vi "getChannelNumber.vi"(8 "error in (no error)":errorcluster, 11 "SoundAO in":refnum<class "SoundAO.lvclass">) -> (0 "error out":errorcluster, 2 "numberOfChannels":i32, 3 "SoundAO out":refnum<class "SoundAO.lvclass">)   [LabVIEW 2009, in "Hardware.lvlib" / "Channels.lvlib" / "SoundAO.lvclass"]
uses:
  SoundAO.lvclass
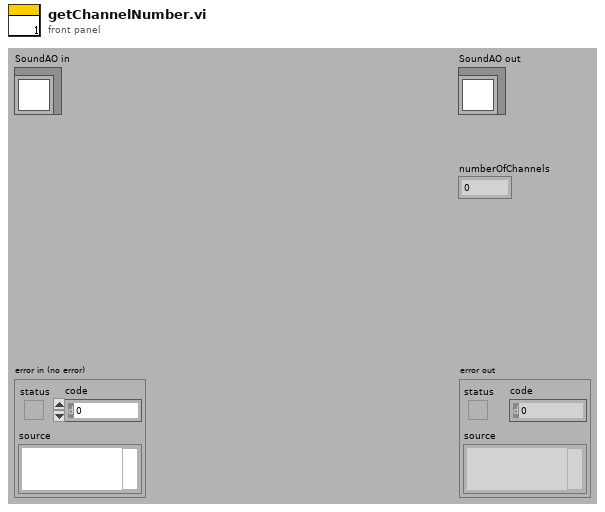
[diagram p1: front panel]
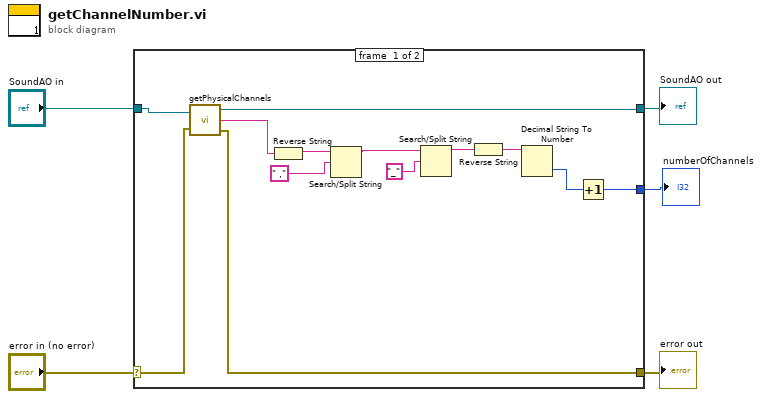
[diagram p0: block diagram]
diagram:
  n1 = case shown="No Error" "error in (no error)" {
    selector: "error in (no error)" -> [w17 w20]
    tunnel: [w15 w20] -> w4
    tunnel: [w16 w19] -> w2
    tunnel: "SoundAO in" -> [w18 w19]
    tunnel: [w6 _] -> w1
    frame #0 {
      n2 = call-dynamic "getPhysicalChannels.vi"("AnalogOutput.lvclass in"=w18, "error in (no error)"=w17) -> ("AnalogOutput.lvclass out"=w16:refnum<class "SoundAO.lvclass">, "Physical Channels"=w14:string, "error out"=w15:errorcluster)
      n3 = Reverse String(1:w14) -> (0:w13:string)
      n4 = Search/Split String(string=w13, search string/char (-)=" ,") -> (substring before match=w10:string)  [unwired: 1 in, 2 out]
      n5 = Search/Split String(string=w10, search string/char (-)="_") -> (substring before match=w7:string)  [unwired: 1 in, 2 out]
      n6 = Reverse String(1:w7) -> (0:w8:string)
      n7 = Decimal String To Number(string=w8) -> (number=w11:i32)  [unwired: 2 in, 1 out]
      n8 = Increment(x=w11) -> (x+1=w6:i32)
    }
    frame #1 {
    }
  }
  "error out" <- w4
  "SoundAO out" <- w2
  "numberOfChannels" <- w1
